vi "Display Image.vi"(7 "Size Mode (Zoom)":enum16{"Normal", "Stretch", "Center", "Zoom"}(ring)=enum."Zoom", 8 "error in (no error)":errorcluster, 10 "Image":refnum<k24>, 11 "PictureBox":refnum<k24>(container)) -> (0 "error out":errorcluster, 3 "PictureBox Out":refnum<k24>)   [LabVIEW 2013]
doc: "This VI will display an <B>Image</B> into the <B>PictureBox</B> using the <B>Size Mode (Zoom)</B> settings. If no Image is passed in, the SizeMode will be applied to the image in the PictureBox and no new image will be loaded.\n\n-----\nBrian Hoover (hooovahh)"
uses:
  System.Windows.Forms
  System.Drawing
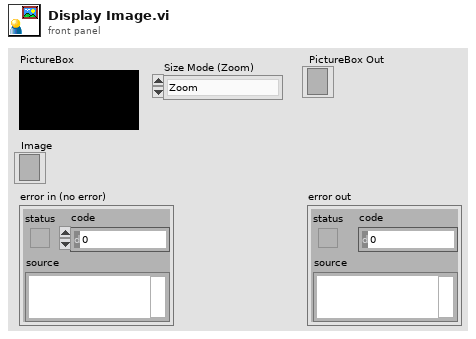
[diagram p1: front panel]
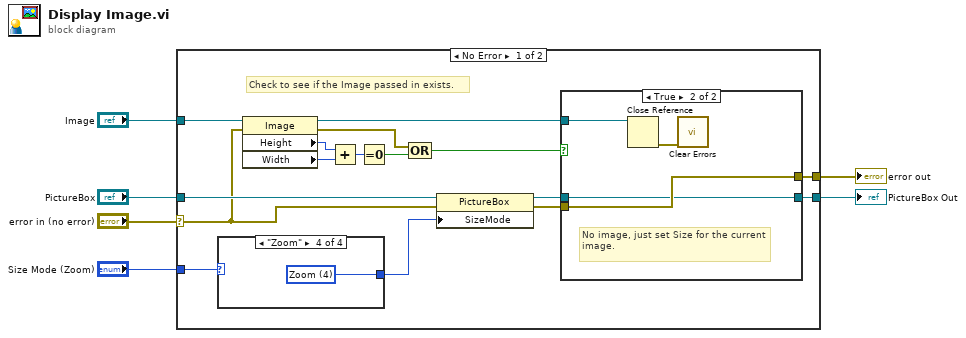
[diagram p0: block diagram]
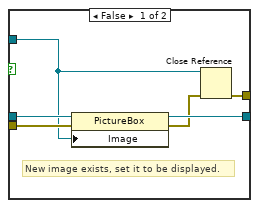
[diagram p2: hidden frame]
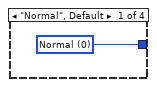
[diagram p3: hidden frame]
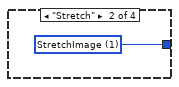
[diagram p4: hidden frame]
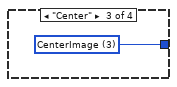
[diagram p5: hidden frame]
diagram:
  n1 = case shown="No Error" "error in (no error)" {
    selector: "error in (no error)" -> [w11 w38]
    tunnel: "Size Mode (Zoom)" -> [w22 _]
    tunnel: "PictureBox" -> [w21 w37]
    tunnel: [w17 w37] -> w4
    tunnel: "Image" -> [w15 _]
    tunnel: [w16 w38] -> w3
    frame No Error {
      # "Check to see if the Image passed in exists."
      n2 = case shown="\"Zoom\"" w22 {
        tunnel: [w33 w34 w35 w36] -> w20
        frame "Normal", Default {
          w33 = 0 items=["Normal", "StretchImage", "AutoSize", "CenterImage", "Zoom"] ("Size Mode (Zoom) 2")
        }
        frame "Stretch" {
          w34 = 1 items=["Normal", "StretchImage", "AutoSize", "CenterImage", "Zoom"] ("Size Mode (Zoom) 2")
        }
        frame "Center" {
          w35 = 3 items=["Normal", "StretchImage", "AutoSize", "CenterImage", "Zoom"] ("Size Mode (Zoom) 2")
        }
        frame "Zoom" {
          w36 = 4 items=["Normal", "StretchImage", "AutoSize", "CenterImage", "Zoom"] ("Size Mode (Zoom) 2")
        }
      }
      n3 = property class="Image"(reference=w15, error in=w11) -> (reference out=w7:refnum<k24>, error out=w9:errorcluster, "Height"=w14:i32, "Width"=w13:i32)
      n4 = Add(x=w14, y=w13) -> (x+y=w12:i32)
      n5 = Equal To 0?(x=w12) -> (x = 0?=w10:bool)
      n6 = Compound Arithmetic op=OR(w9, w10) -> (w8:bool)
      n7 = property class="PictureBox"(reference=w21, error in=w11, "SizeMode"=w20) -> (reference out=w19:refnum<k24>, error out=w18:errorcluster)
      n8 = case shown="True" w8 {
        tunnel: w19 -> [w28 w31]
        tunnel: w18 -> [w27 w32]
        tunnel: [w26 w31] -> w17
        tunnel: [w24 w32] -> w16
        tunnel: w7 -> [w23 w30]
        frame False {
          # "New image exists, set it to be displayed."
          n9 = property class="PictureBox"(reference=w28, error in=w27, "Image"=w23) -> (reference out=w26:refnum<k24>, error out=w25:errorcluster)
          n10 = Close Reference(reference=w23, error in (no error)=w25) -> (error out=w24:errorcluster)
        }
        frame True {
          # "No image, just set Size for the current image."
          n11 = Close Reference(reference=w30) -> (error out=w29:errorcluster)  [unwired: 1 in]
          n12 = call <vilib>:"Clear Errors.vi"("error in (no error)"=w29) -> ()  [unwired: 6 in, 1 out]
        }
      }
    }
    frame Error {
    }
  }
  "PictureBox Out" <- w4
  "error out" <- w3
